vi "Is equal in tolerance.vi"(1 "Absolut tolerance":dbl, 2 "Reference value":dbl, 4 "Input value":dbl) -> (0 "Is in range":bool)   [LabVIEW 2017, in "Magnet module.lvlib"]
doc: "Check if input value is in tolerance range with reference values."
uses:
  Magnet module.lvlib
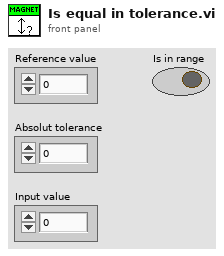
[diagram p1: front panel]
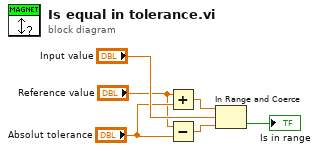
[diagram p0: block diagram]
diagram:
  n1 = Add(x="Reference value", y="Absolut tolerance") -> (x+y=w3:dbl)
  n2 = Subtract(x="Reference value", y="Absolut tolerance") -> (x-y=w2:dbl)
  n3 = In Range and Coerce(upper limit=w3, x="Input value", lower limit=w2) -> (In Range?=→"Is in range":bool)  [unwired: 1 out]
